vi "test match multiple pattern.vi"() -> ()   [LabVIEW 2017]
panel:
  out "pattern matched":string
  out "Found?":bool
  out "match substring":string
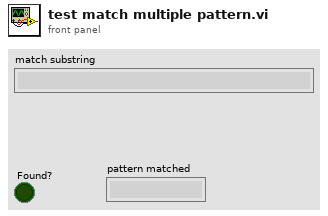
[diagram p1: front panel]
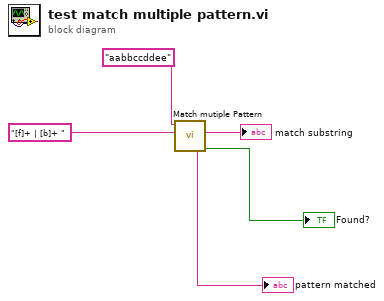
[diagram p0: block diagram]
diagram:
  n1 = call "Match mutiple Pattern.vi"("regular expression"="[f]+ | [b]+ ", "string"="aabbccddee") -> ("Found?"=→"Found?":bool, "match substring"=→"match substring":string, "pattern matched"=→"pattern matched":string)  [unwired: 5 in, 2 out]
